vi "LVSPrtHlp.vi"(11 "VISA resource name":refnum<visa-resource-name>) -> (0 "error?":bool, 2 "string read":string)   [LabVIEW 2013]
uses:
  instr.lib/lvserial/lvserial.lvlib
  <vilib>/Utility/error.llb/DialogType.ctl
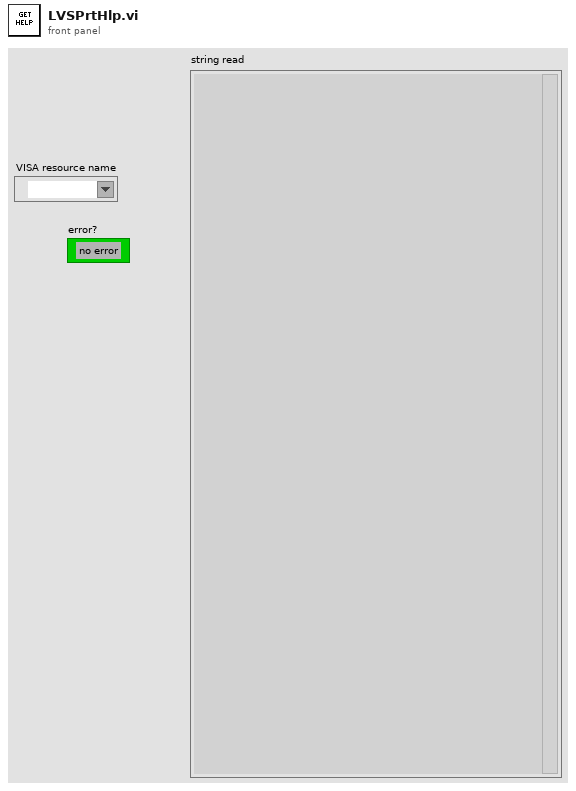
[diagram p1: front panel]
types:
  T1 = typedef "DialogType.ctl" = u16
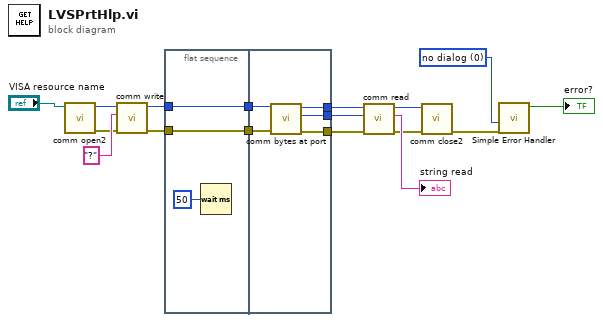
[diagram p0: block diagram]
diagram:
  w3 = T1 0 items=["no dialog", "OK message", "continue or stop message", "OK message + warnings", "continue/stop + warnings"] ("type of dialog (OK msg:1)")
  n1 = call "comm open2.vi"("Comm Port Name"="VISA resource name") -> ("error out"=w13:errorcluster, "Comm Handle"=w12:u32)  [unwired: 4 in, 1 out]
  n2 = call "comm write.vi"("error in (no error)"=w13, "string to write"="?", "Comm Handle"=w12) -> ("error out"=w7:errorcluster, "dup Comm Handle"=w8:u32)  [unwired: 6 in, 1 out]
  n3 = flat-sequence {
    tunnel: w8 -> [w19]
    tunnel: w7 -> [w18]
    tunnel: [w19] -> w10
    tunnel: [w18] -> w9
    tunnel: [w25] -> w11
    tunnel: w10 -> [w24]
    tunnel: w9 -> [w23]
    tunnel: [w22] -> w5
    tunnel: [w21] -> w4
    frame #0 {
      n4 = Wait (ms)(milliseconds to wait=u32 50) -> ()  [unwired: 1 out]
    }
    frame #1 {
      n5 = call "comm bytes at port.vi"("error in (no error)"=w23, "Comm Handle"=w24) -> ("error out"=w21:errorcluster, "bytes at port"=w25:u32, "dup Comm Handle"=w22:u32)  [unwired: 7 in]
    }
  }
  n6 = call "comm read.vi"("error in (no error)"=w4, "requested byte count"=w11, "Comm Handle"=w5) -> ("error out"=w6:errorcluster, "string read"=→"string read":string, "dup Comm Handle"=w16:u32)  [unwired: 5 in, 1 out]
  n7 = call "comm close2.vi"("error in (no error)"=w6, "Comm Handle"=w16) -> ("error out"=w1:errorcluster)  [unwired: 5 in]
  n8 = call <vilib>:"Simple Error Handler.vi"("type of dialog (OK msg:1)"=w3, "error in (no error)"=w1) -> ("error?"=→"error?":bool)  [unwired: 7 out]
